vi "LINX - Test Leds with servo.vi"() -> ()   [LabVIEW 2019]
doc: "Manually blink and LED attached to a digital output channel of a LINX device by clicking and LED control in LabVIEW."
uses:
  <vilib>/MakerHub/LINX/Public/Utilities/Open Serial.vi
  <vilib>/MakerHub/LINX/Public/Sensors/Motion/Servo/Servo Open One Channel.vi
  <vilib>/MakerHub/LINX/Public/Sensors/Motion/Servo/Servo Set Pulse Width One Channel.vi
  <vilib>/MakerHub/LINX/Public/Peripherals/Digital/Digital Write N Chans.vi
  <vilib>/MakerHub/LINX/LMH-LINX.lvlib
  <vilib>/MakerHub/LINX/Public/Sensors/Motion/Servo/Servo.lvlib
panel:
  in  "Cerrar":bool
  in  "Abrir":bool
  in  "Servo Channel":u8=2
  in  "Values":bool[](array[boolean])
  in  "DO Channels":u8[](array[numeric])
  out "Loop Rate (Hz)":u32
  in  "Serial Port":refnum<visa-resource-name>
  in  "Stop Button":bool
  # "Circuit Schematic"
  # "LINX Device Settings"
  # "LED Control"
  # "BOTON VERDE"
  # "BOTON ROJO"
  # "^^ Click Here ^^"
  # "Manual Blink Example\n\nThis example demonstrates how to blink an LED on a LINX device by clicking on an LED control in LabVIEW.\n\nInstructions\n1. Select the Serial Port associated with the LINX Device.\n2. Select the Digital Output Channel connected to the LED.\n3. Click the Run Arrow."
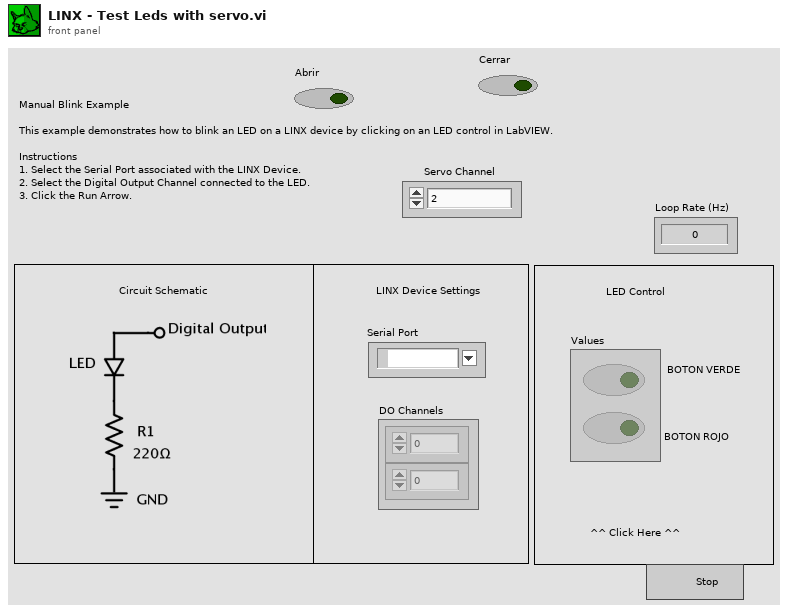
[diagram p1: front panel]
types:
  T1 = typedef "LMH-LINX.lvlib/LINX Ref.ctl" = cluster{"IO":T2, "Interface":T3, "LINX Device Config":T4}
  T2 = typedef "LMH-LINX.lvlib/Platform.ctl" = enum16{"Remote", "Local"}
  T3 = typedef "LMH-LINX.lvlib/Interface.ctl" = enum16{"Serial", "TCP"}
  T4 = typedef "LMH-LINX.lvlib/Device.lvlib/LINX Device Config.ctl" = cluster{"Interface":T3, "COM Port":refnum<visa-resource-name>, "TCP Configuration":T5, "Device Family":u8, "Device ID":u8, "Device Name":string, "TCP Ref":refnum<k5>, "Channels":T6}
  T5 = typedef "LMH-LINX.lvlib/Device.lvlib/TCP Config.ctl" = cluster{"IP Address":string, "Port":u16}
  T6 = typedef "LMH-LINX.lvlib/Channels.ctl" = cluster{"DI":u8[], "DO":u8[], "AI":u8[], "AO":u8[], "PWM":u8[], "QE":u8[], "UART":u8[], "I2C 2":u8[], "SPI":u8[], "CAN":u8[], "Servo":u8[], "AI Ref (V)":dbl, "AI Resolution (Bits)":u8, "AO Ref (V)":dbl, "AO Resolution (Bits)":u8}
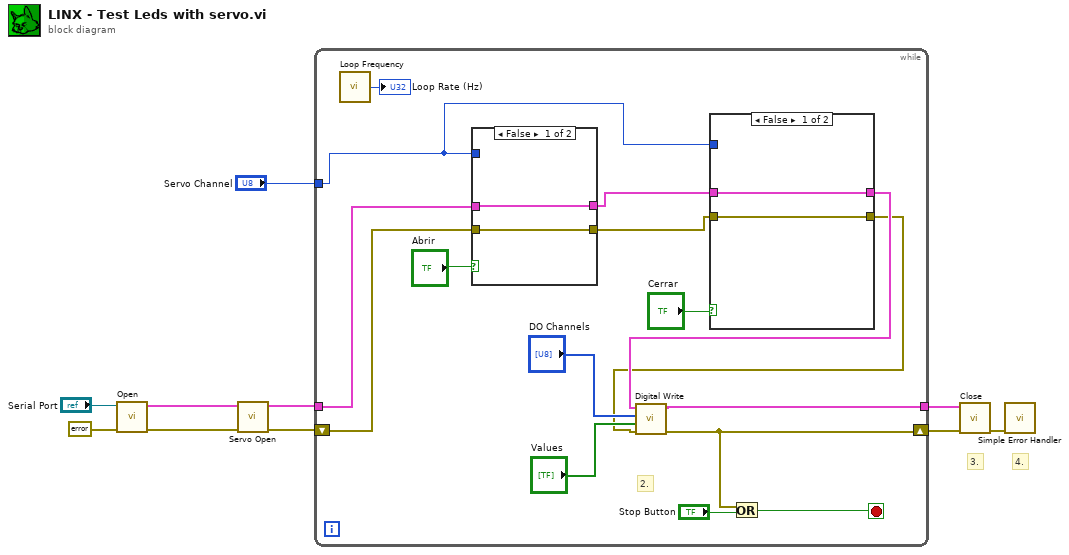
[diagram p0: block diagram]
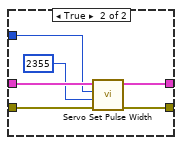
[diagram p2: hidden frame]
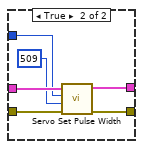
[diagram p3: hidden frame]
diagram:
  # "4."
  # "3."
  n1 = call-poly <vilib>:"Open.vi"("Error In"=errorcluster {"status"=FALSE, "code"=0, "source"=""}, "Serial Port"="Serial Port") -> ("Error Out"=w3:errorcluster, "LINX Resource"=w4:T1)  [unwired: 7 in, 1 out]
  n2 = call-poly <vilib>:"Servo Open.vi"("Error In"=w3, "LINX Resource"=w4) -> ("Error Out"=w1:errorcluster, "LINX Resource"=w2:T1)  [unwired: 8 in]
  n3 = while {
    tunnel: w2 -> [w18]
    tunnel: [w24] -> w10
    shift-right: [w23] -> w9
    shift-left: w1 -> [w17]
    tunnel: "Servo Channel" -> [w13]
    stop <- w26 stop-if-true
    # "2."
    n4 = call <vilib>:"Loop Frequency.vi"() -> ("Loop Rate (Hz)"=→"Loop Rate (Hz)":u32)
    n5 = case shown="False" "Abrir" {
      tunnel: w17 -> [w35 w42]
      tunnel: [w35 w41] -> w15
      tunnel: w18 -> [w36 w40]
      tunnel: [w36 w39] -> w14
      tunnel: w13 -> [_ w38]
      frame False {
      }
      frame True {
        n6 = call-poly <vilib>:"Servo Set Pulse Width.vi"("Error In"=w42, "Pulse Width (uS)"=509, "Servo Channel"=w38, "LINX Resource"=w40) -> ("Error Out"=w41:errorcluster, "LINX Resource"=w39:T1)  [unwired: 6 in]
      }
    }
    n7 = case shown="False" "Cerrar" {
      tunnel: w15 -> [w27 w34]
      tunnel: [w27 w33] -> w11
      tunnel: w14 -> [w28 w32]
      tunnel: [w28 w31] -> w12
      tunnel: w13 -> [_ w30]
      frame False {
      }
      frame True {
        n8 = call-poly <vilib>:"Servo Set Pulse Width.vi"("Error In"=w34, "Pulse Width (uS)"=2355, "Servo Channel"=w30, "LINX Resource"=w32) -> ("Error Out"=w33:errorcluster, "LINX Resource"=w31:T1)  [unwired: 6 in]
      }
    }
    n9 = call-poly <vilib>:"Digital Write.vi"("Error In"=w11, "Values"="Values", "DO Channels"="DO Channels", "LINX Resource"=w12) -> ("Error Out"=w23:errorcluster, "LINX Resource"=w24:T1)  [unwired: 6 in]
    n10 = Or(x=w23, y="Stop Button") -> (x .or. y?=w26:bool)
  }
  n11 = call <vilib>:"Close.vi"("Error In"=w9, "LINX Resource"=w10) -> ("Error Out"=w7:errorcluster)  [unwired: 9 in]
  n12 = call <vilib>:"Simple Error Handler.vi"("error in (no error)"=w7) -> ()  [unwired: 4 in, 5 out]
